vi "Update Dashboard Display Objects.vi"(8 "Error In":errorcluster, 11 "Display Manager In":refnum<class "Display Manager.lvclass">) -> (0 "Error Out":errorcluster, 3 "Display Manager Out":refnum<class "Display Manager.lvclass">)   [LabVIEW 2019, in "Display Manager.lvclass"]
uses:
  Display Manager.lvclass
  <vilib>/Memosfet/myRIO-Neopixel/RT/String/String.lvclass
  Accessors/Display/Get Display.vi
  <vilib>/Memosfet/myRIO-Neopixel/RT/Display/Display.lvclass
  <vilib>/Memosfet/myRIO-Neopixel/RT/Display Element/Display Element.lvclass
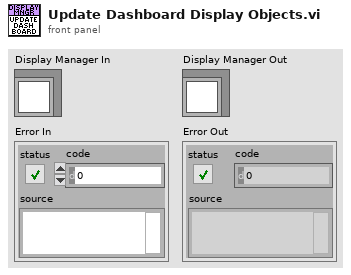
[diagram p1: front panel]
types:
  T1 = typedef "LVDateTimeRec.ctl" = cluster{"fractional second":dbl, "second":i32, "minute":i32, "hour":i32, "day of month":i32, "month":i32, "year":i32, "day of week":i32, "day of year":i32, "DST":i32}
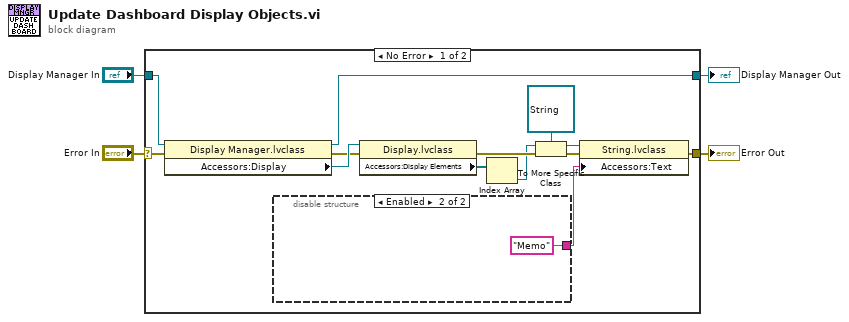
[diagram p0: block diagram]
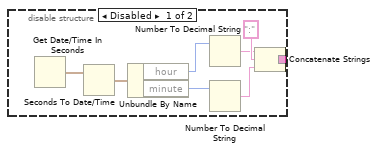
[diagram p2: hidden frame]
diagram:
  n1 = case shown="No Error" "Error In" {
    selector: "Error In" -> [w16 w28]
    tunnel: [w14 w28] -> w3
    tunnel: "Display Manager In" -> [w17 w27]
    tunnel: [w15 w27] -> w1
    frame No Error {
      n2 = property class="Display Manager.lvclass"(reference=w17, error in=w16) -> (reference out=w15:refnum<class "Display Manager.lvclass">, error out=w12:errorcluster, "Accessors:Display"=w13:refnum<class "Display.lvclass">)
      n3 = disable-structure shown="Enabled" {
        disable-tunnel: [w18 "Memo"] -> w5
        frame Disabled {
          n4 = Get Date/Time In Seconds() -> (seconds since 1Jan1904=w25:timestamp)
          n5 = Seconds To Date/Time(time stamp (now)=w25) -> (date time rec=w24:T1)  [unwired: 1 in]
          n6 = Unbundle By Name(w24) -> ("hour"=w22:i32, "minute"=w21:i32)
          n7 = Number To Decimal String(number=w22) -> (decimal integer string=w19:string)  [unwired: 1 in]
          n8 = Number To Decimal String(number=w21) -> (decimal integer string=w23:string)  [unwired: 1 in]
          n9 = Concatenate Strings(w19, ":" ("string"), w23) -> (w18:string)
        }
        frame Enabled {
        }
      }
      n10 = property class="Display.lvclass"(reference=w13, error in=w12) -> (error out=w10:errorcluster, "Accessors:Display Elements"=w11:refnum<class "Display Element.lvclass">[])  [unwired: 1 out]
      n11 = Index Array(array=w11) -> (element=w9:refnum<class "Display Element.lvclass">)  [unwired: 1 in]
      n12 = To More Specific Class(target class=refnum<class "String.lvclass"> refnum ("Pixel In"), reference=w9, error in=w10) -> (specific class reference=w7:refnum<class "String.lvclass">, error out=w6:errorcluster)
      n13 = property class="String.lvclass"(reference=w7, error in=w6, "Accessors:Text"=w5) -> (error out=w14:errorcluster)  [unwired: 1 out]
    }
    frame Error {
    }
  }
  "Display Manager Out" <- w1
  "Error Out" <- w3
